vi "XiXi-1(Divide DBL).vi"(10 "X[-1]":dbl, 11 "Xi":dbl[](array[numeric])) -> (2 "Remain":dbl[](array[numeric]) format="%.2f", 3 "Yi":dbl[](array[numeric]) format="%.2f")   [LabVIEW 2012]
doc: "Calculate sums of consecutive array elements. 0th element of output is equal to x(0)+ x(-1), where x(-1) is an optional scalar input that defaults to zero."
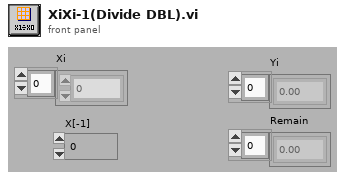
[diagram p1: front panel]
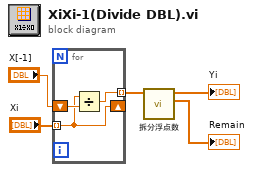
[diagram p0: block diagram]
diagram:
  n1 = for {
    shift-right: [w7] -> _
    shift-left: "X[-1]" -> [w8]
    tunnel: "Xi" -> [w7] mode=indexing
    tunnel: [w6] -> w1 mode=indexing
    n2 = Divide(x=w7, y=w8) -> (x/y=w6:dbl)
  }
  n3 = call-poly "拆分浮点数.vi"("输入"=w1) -> ("小数部分"=→"Remain":dbl[], "整数部分"=→"Yi":dbl[])  [unwired: 9 in]
